vi "GetBlock.vi"(0 "error in":errorcluster, 2 "handle in":i16, 3 "Acquisition Settings":T3={"preTriggerSamples"=0, "postTriggerSamples"=1000, "timebase"=2, "Down-Sample Mode"=0, "Down Sample Ratio"=1} {"Down Sample Ratio" min=1 step=1; "Down-Sample Mode" items=["None"=0, "Aggregate"=1, "Decimate"=2, "Average"=4]}, 5 "enabled array":i16[](array[numeric])) -> (4 "overflow":i16, 6 "error IO":errorcluster, 7 "handle out":i16, 8 "noOfSamples":u32, 9 "Buffers (Max or non-aggregated)":T1, 10 "Min Buffers":T2)   [LabVIEW 2017]
doc: "This VI collects a block of data from the oscilloscope. This can be called in a loop in order to continually collect blocks of data. The oscilloscope should first be set up by using PicoScope3000aSettings.vi. The VI outputs data arrays in two clusters (max and min). If not using aggregation, 'Min Buffers' is not used."
uses:
  ps5000a.dll
panel:
  out "32bit integer":i32
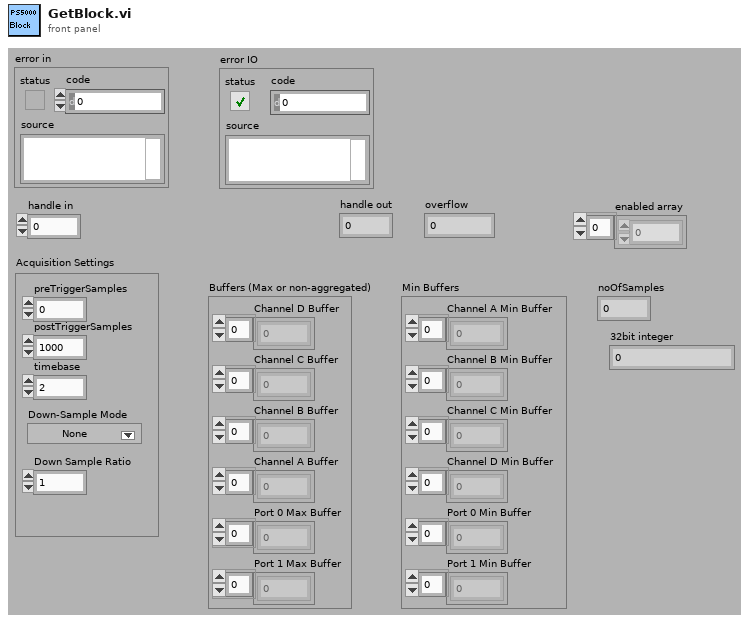
[diagram p1: front panel]
types:
  T1 = cluster{"Channel D Buffer":i16[], "Channel C Buffer":i16[], "Channel B Buffer":i16[], "Channel A Buffer":i16[], "Port 0 Max Buffer":i32[], "Port 1 Max Buffer":i32[]}
  T2 = cluster{"Channel A Min Buffer":i16[], "Channel B Min Buffer":i16[], "Channel C Min Buffer":i16[], "Channel D Min Buffer":i16[], "Port 0 Min Buffer":i32[], "Port 1 Min Buffer":i32[]}
  T3 = cluster{"preTriggerSamples":i32, "postTriggerSamples":i32, "timebase":u32, "Down-Sample Mode":u32, "Down Sample Ratio":u32}
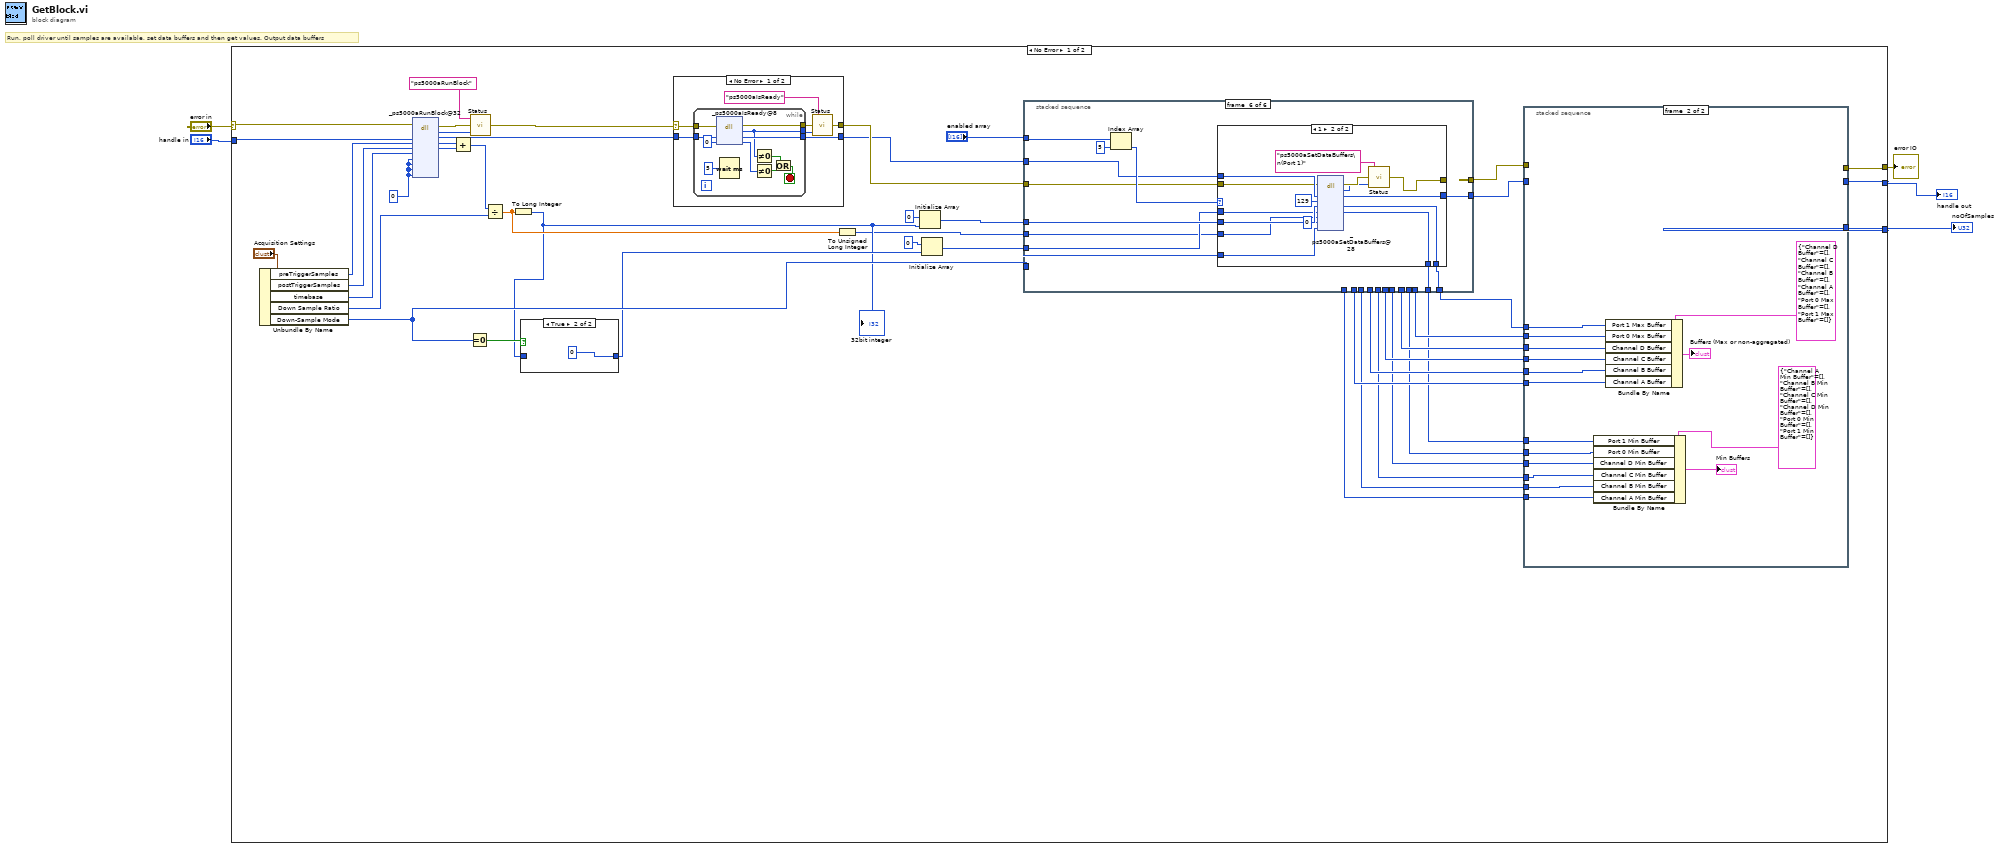
[diagram p0: block diagram]
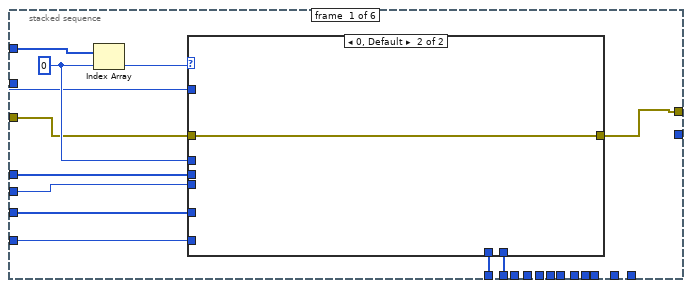
[diagram p3: hidden frame]
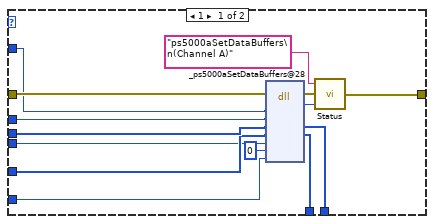
[diagram p4: hidden frame]
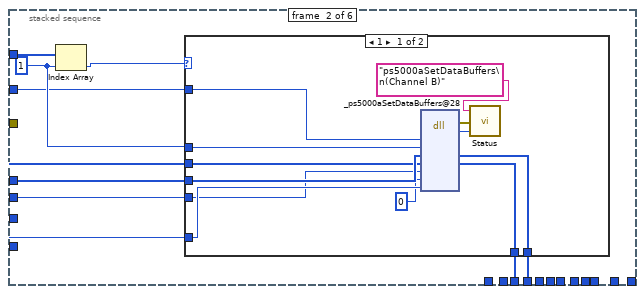
[diagram p5: hidden frame]
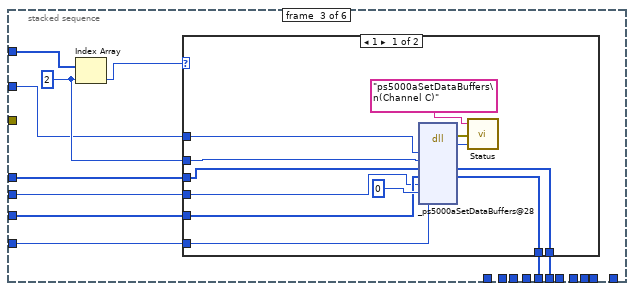
[diagram p7: hidden frame]
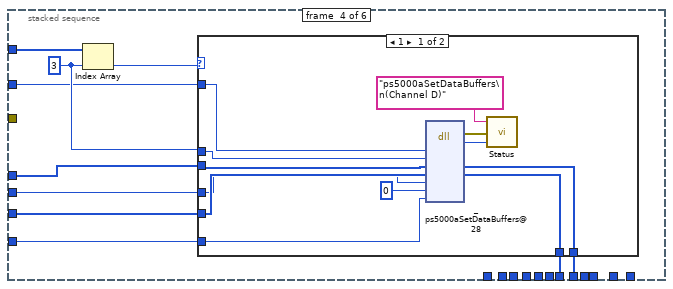
[diagram p9: hidden frame]
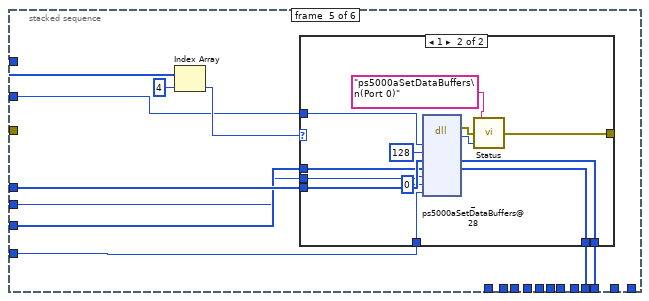
[diagram p11: hidden frame]
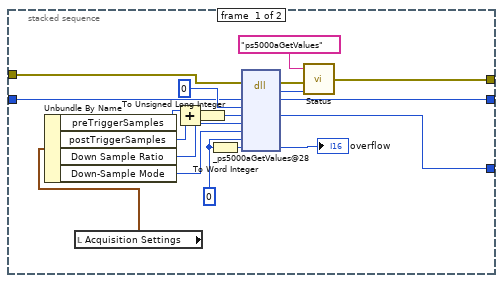
[diagram p14: hidden frame]
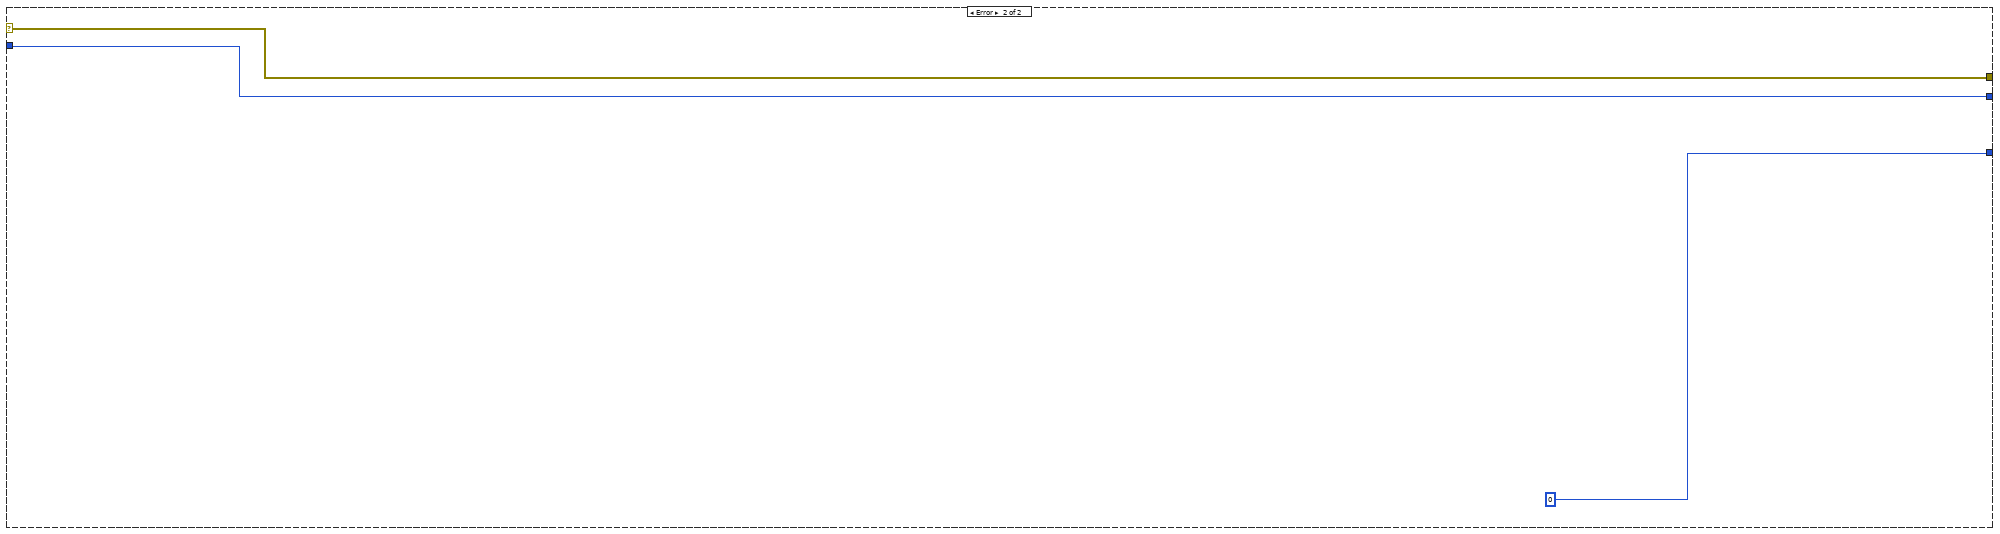
[diagram p16: hidden frame]
diagram:
  # "Run, poll driver until samples are available, set data buffers and then get values. Output data buffers"
  n1 = case shown="No Error" "error in" {
    selector: "error in" -> [w45 w255]
    tunnel: [w6 w255] -> w1
    tunnel: "handle in" -> [w44 w254]
    tunnel: [w43 w254] -> w5
    tunnel: [w36 u32 0 ("noOfSamples")] -> w2
    frame No Error {
      w40 = u32 0 ("pParameter")
      n2 = Unbundle By Name("Acquisition Settings") -> ("preTriggerSamples"=w39:i32, "postTriggerSamples"=w38:i32, "timebase"=w37:u32, "Down Sample Ratio"=w41:u32, "Down-Sample Mode"=w26:u32)
      n3 = dll-call lib="ps5000a.dll" fn="_ps5000aRunBlock@32" ("ps3000.dll:_ps3000_open_unit@0")(error in=w45, "handle"=w44, "preTriggerSamples"=w39, "postTriggerSamples"=w38, "timebase"=w37, "timeindisposed"=w40, "segmentIndex"=w40, "lpReady"=w40, "pParameter"=w40) -> (error out=w47:errorcluster, "PICO_STATUS"=w48:u32, "handle"=w35:i16, "preTriggerSamples"=w51:i32, "postTriggerSamples"=w50:i32)  [unwired: 7 in, 1 out]
      n4 = Add(x=w51, y=w50) -> (x+y=w42:i32)
      n5 = Equal To 0?(x=w26) -> (x = 0?=w24:bool)
      n6 = call "Status.vi"("PICO STATUS"=w48, "error in"=w47, "source"="ps5000aRunBlock") -> ("error out"=w7:errorcluster)
      n7 = Divide(x=w42, y=w41) -> (x/y=w27:dbl)
      n8 = To Long Integer(number=w27) -> (32bit integer=w23:i32)
      "32bit integer" <- w23
      n9 = case shown="True" w24 {
        tunnel: [w52 0] -> w25
        tunnel: w23 -> [w52 _]
        frame False {
        }
        frame True {
        }
      }
      n10 = case shown="No Error" w7 {
        selector: w7 -> [w237 w251]
        tunnel: w35 -> [w239 w252]
        tunnel: [w238 w252] -> w30
        tunnel: [w236 w251] -> w31
        frame No Error {
          n11 = while {
            tunnel: [w250] -> w238
            tunnel: w239 -> [w249]
            tunnel: [w244] -> w234
            tunnel: w237 -> [w243]
            tunnel: [w242] -> w235
            stop <- w248 stop-if-true
            n12 = dll-call lib="ps5000a.dll" fn="_ps5000aIsReady@8" ("ps3000.dll:_ps3000_open_unit@0")(error in=w243, "handle"=w249, "ready"=i16 0) -> (error out=w242:errorcluster, "PICO_STATUS"=w244:u32, "handle"=w250:i16, "ready"=w245:i16)  [unwired: 2 in, 1 out]
            n13 = Wait (ms)(milliseconds to wait=5) -> ()  [unwired: 1 out]
            n14 = Not Equal To 0?(x=w244) -> (x != 0?=w246:bool)
            n15 = Not Equal To 0?(x=w245) -> (x != 0?=w247:bool)
            n16 = Or(x=w246, y=w247) -> (x .or. y?=w248:bool)
          }
          n17 = call "Status.vi"("PICO STATUS"=w234, "error in"=w235, "source"="ps5000aIsReady") -> ("error out"=w236:errorcluster)
        }
        frame Error {
        }
      }
      n18 = To Unsigned Long Integer(number=w27) -> (unsigned 32bit integer=w9:u32)
      n19 = Initialize Array(i16 0 ("element"), w23) -> (w29:i16[])
      n20 = Initialize Array(i16 0 ("element"), w25) -> (w28:i16[])
      n21 = stacked-sequence {
        tunnel: "enabled array" -> [w64 w88 w111 w132 w156 w181]
        tunnel: w31 -> [w62 _ _ _ _ w170]
        tunnel: w30 -> [w61 w87 w109 w131 w153 w178]
        tunnel: w29 -> [w60 w86 w108 w130 w152 w177]
        tunnel: w28 -> [w59 w85 w107 w129 w151 w176]
        tunnel: w9 -> [w58 w83 w106 w128 w150 w175]
        tunnel: w26 -> [w57 w84 w105 w127 w149 w174]
        tunnel: [w56 _ _ _ _ _] -> w22
        tunnel: [w55 _ _ _ _ _] -> w21
        tunnel: [_ w82 _ _ _ _] -> w20
        tunnel: [_ w81 _ _ _ _] -> w19
        tunnel: [_ _ w104 _ _ _] -> w18
        tunnel: [_ _ w103 _ _ _] -> w17
        tunnel: [_ _ _ w126 _ _] -> w16
        tunnel: [_ _ _ w125 _ _] -> w15
        tunnel: [_ _ _ _ w148 _] -> w14
        tunnel: [_ _ _ _ w147 _] -> w13
        tunnel: [_ _ _ _ _ w173] -> w12
        tunnel: [_ _ _ _ _ w172] -> w11
        tunnel: [w54 _ _ _ _ _] -> w10
        tunnel: [_ _ _ _ _ w171] -> w8
        frame #0 {
          w65 = 0 ("dimension size")
          n22 = Index Array(array=w64, index=w65) -> (element=w63:i16)
          n23 = case shown="0, Default" w63 {
            tunnel: w65 -> [w74 _]
            tunnel: w62 -> [w79 w80]
            tunnel: w61 -> [w76 _]
            tunnel: w60 -> [w73 _]
            tunnel: w59 -> [w72 _]
            tunnel: w58 -> [w71 _]
            tunnel: w57 -> [w70 _]
            tunnel: [w68 _] -> w56
            tunnel: [w67 _] -> w55
            tunnel: [w66 w80] -> w54
            frame 1 {
              n24 = dll-call lib="ps5000a.dll" fn="_ps5000aSetDataBuffers@28" ("ps3000.dll:_ps3000_open_unit@0")(error in=w79, "handle"=w76, "channel"=w74, "bufferMax"=w73, "bufferMin"=w72, "bufferLth"=w71, "segmentIndex"=u32 0, "mode"=w70) -> (error out=w78:errorcluster, "PICO_STATUS"=w77:u32, "bufferMax"=w67:i16[], "bufferMin"=w68:i16[])  [unwired: 7 in, 1 out]
              n25 = call "Status.vi"("PICO STATUS"=w77, "error in"=w78, "source"="ps5000aSetDataBuffers\n(Channel A)") -> ("error out"=w66:errorcluster)
            }
            frame 0, Default {
            }
          }
        }
        frame #1 {
          w90 = 1 ("dimension size")
          n26 = Index Array(array=w88, index=w90) -> (element=w89:i16)
          n27 = case shown="1" w89 {
            tunnel: w90 -> [w99 _]
            tunnel: w87 -> [w98 _]
            tunnel: w86 -> [w97 _]
            tunnel: w85 -> [w96 _]
            tunnel: w84 -> [w95 _]
            tunnel: w83 -> [w93 _]
            tunnel: [w92 _] -> w82
            tunnel: [w91 _] -> w81
            frame 1 {
              n28 = dll-call lib="ps5000a.dll" fn="_ps5000aSetDataBuffers@28" ("ps3000.dll:_ps3000_open_unit@0")("handle"=w98, "channel"=w99, "bufferMax"=w97, "bufferMin"=w96, "bufferLth"=w93, "segmentIndex"=u32 0, "mode"=w95) -> (error out=w101:errorcluster, "PICO_STATUS"=w102:u32, "bufferMax"=w91:i16[], "bufferMin"=w92:i16[])  [unwired: 8 in, 1 out]
              n29 = call "Status.vi"("PICO STATUS"=w102, "error in"=w101, "source"="ps5000aSetDataBuffers\n(Channel B)") -> ()  [unwired: 1 out]
            }
            frame 0, Default {
            }
          }
        }
        frame #2 {
          w112 = 2 ("dimension size")
          n30 = Index Array(array=w111, index=w112) -> (element=w110:i16)
          n31 = case shown="1" w110 {
            tunnel: w112 -> [w120 _]
            tunnel: w109 -> [w119 _]
            tunnel: w108 -> [w118 _]
            tunnel: w107 -> [w117 _]
            tunnel: w106 -> [w116 _]
            tunnel: w105 -> [w115 _]
            tunnel: [w114 _] -> w104
            tunnel: [w113 _] -> w103
            frame 1 {
              n32 = dll-call lib="ps5000a.dll" fn="_ps5000aSetDataBuffers@28" ("ps3000.dll:_ps3000_open_unit@0")("handle"=w119, "channel"=w120, "bufferMax"=w118, "bufferMin"=w117, "bufferLth"=w116, "segmentIndex"=u32 0, "mode"=w115) -> (error out=w123:errorcluster, "PICO_STATUS"=w124:u32, "bufferMax"=w113:i16[], "bufferMin"=w114:i16[])  [unwired: 8 in, 1 out]
              n33 = call "Status.vi"("PICO STATUS"=w124, "error in"=w123, "source"="ps5000aSetDataBuffers\n(Channel C)") -> ()  [unwired: 1 out]
            }
            frame 0, Default {
            }
          }
        }
        frame #3 {
          w134 = 3 ("dimension size")
          n34 = Index Array(array=w132, index=w134) -> (element=w133:i16)
          n35 = case shown="1" w133 {
            tunnel: w134 -> [w142 _]
            tunnel: w131 -> [w141 _]
            tunnel: w130 -> [w140 _]
            tunnel: w129 -> [w139 _]
            tunnel: w128 -> [w138 _]
            tunnel: w127 -> [w137 _]
            tunnel: [w136 _] -> w126
            tunnel: [w135 _] -> w125
            frame 1 {
              n36 = dll-call lib="ps5000a.dll" fn="_ps5000aSetDataBuffers@28" ("ps3000.dll:_ps3000_open_unit@0")("handle"=w141, "channel"=w142, "bufferMax"=w140, "bufferMin"=w139, "bufferLth"=w138, "segmentIndex"=u32 0, "mode"=w137) -> (error out=w145:errorcluster, "PICO_STATUS"=w146:u32, "bufferMax"=w135:i16[], "bufferMin"=w136:i16[])  [unwired: 8 in, 1 out]
              n37 = call "Status.vi"("PICO STATUS"=w146, "error in"=w145, "source"="ps5000aSetDataBuffers\n(Channel D)") -> ()  [unwired: 1 out]
            }
            frame 0, Default {
            }
          }
        }
        frame #4 {
          n38 = Index Array(array=w156, index=4) -> (element=w154:i16)
          n39 = case shown="1" w154 {
            tunnel: w153 -> [_ w165]
            tunnel: w152 -> [_ w164]
            tunnel: w151 -> [_ w163]
            tunnel: w150 -> [_ w162]
            tunnel: w149 -> [_ w160]
            tunnel: [_ w159] -> w148
            tunnel: [_ w158] -> w147
            tunnel: [_ w157] -> _
            frame 0, Default {
            }
            frame 1 {
              n40 = dll-call lib="ps5000a.dll" fn="_ps5000aSetDataBuffers@28"("handle"=w165, "channel"=128, "bufferMax"=w164, "bufferMin"=w163, "bufferLth"=w162, "segmentIndex"=u32 0, "mode"=w160) -> (error out=w168:errorcluster, "PICO_STATUS"=w169:u32, "bufferMax"=w158:i16[], "bufferMin"=w159:i16[])  [unwired: 8 in, 1 out]
              n41 = call "Status.vi"("PICO STATUS"=w169, "error in"=w168, "source"="ps5000aSetDataBuffers\n(Port 0)") -> ("error out"=w157:errorcluster)
            }
          }
        }
        frame #5 {
          n42 = Index Array(array=w181, index=5) -> (element=w180:i16)
          n43 = case shown="1" w180 {
            tunnel: w178 -> [w182 w194]
            tunnel: w177 -> [_ w193]
            tunnel: w176 -> [_ w192]
            tunnel: w175 -> [_ w191]
            tunnel: w174 -> [_ w189]
            tunnel: [_ w188] -> w173
            tunnel: [_ w187] -> w172
            tunnel: [_ w184] -> _
            tunnel: [w182 w185] -> w171
            tunnel: w170 -> [_ w183]
            frame 0, Default {
            }
            frame 1 {
              n44 = dll-call lib="ps5000a.dll" fn="_ps5000aSetDataBuffers@28" ("ps3000.dll:_ps3000_open_unit@0")(error in=w183, "handle"=w194, "channel"=129, "bufferMax"=w193, "bufferMin"=w192, "bufferLth"=w191, "segmentIndex"=u32 0, "mode"=w189) -> (error out=w197:errorcluster, "PICO_STATUS"=w186:u32, "handle"=w185:i16, "bufferMax"=w187:i16[], "bufferMin"=w188:i16[])  [unwired: 6 in, 1 out]
              n45 = call "Status.vi"("PICO STATUS"=w186, "error in"=w197, "source"="ps5000aSetDataBuffers\n(Port 1)") -> ("error out"=w184:errorcluster)
            }
          }
        }
      }
      n46 = stacked-sequence {
        tunnel: [w211 _] -> w43
        tunnel: [w201 _] -> w36
        tunnel: w22 -> [_ w228]
        tunnel: w21 -> [_ w227]
        tunnel: w20 -> [_ w226]
        tunnel: w19 -> [_ w225]
        tunnel: w18 -> [_ w223]
        tunnel: w17 -> [_ w224]
        tunnel: w16 -> [_ w222]
        tunnel: w15 -> [_ w221]
        tunnel: w14 -> [_ w220]
        tunnel: w13 -> [_ w219]
        tunnel: w12 -> [_ w218]
        tunnel: w11 -> [_ w217]
        tunnel: w10 -> [w200 _]
        tunnel: w8 -> [w199 _]
        tunnel: [w198 _] -> w6
        frame #0 {
          w215 = u32 0 ("overflow")
          n47 = local read "Acquisition Settings"() -> (w209:T3)
          n48 = Unbundle By Name(w209) -> ("preTriggerSamples"=w206:i32, "postTriggerSamples"=w207:i32, "Down Sample Ratio"=w208:u32, "Down-Sample Mode"=w204:u32)
          n49 = Add(x=w206, y=w207) -> (x+y=w205:i32)
          n50 = To Unsigned Long Integer(number=w205) -> (unsigned 32bit integer=w203:u32)
          n51 = To Word Integer(number=w215) -> (16bit integer=w202:i16)
          n52 = dll-call lib="ps5000a.dll" fn="_ps5000aGetValues@28" ("ps3000.dll:_ps3000_open_unit@0")(error in=w200, "handle"=w199, "startIndex"=u32 0, "noOfSamples"=w203, "downSampleRatio"=w208, "downSampleRatioMode"=w204, "segmentIndex"=w215, "overflow"=w202) -> (error out=w213:errorcluster, "PICO_STATUS"=w214:u32, "handle"=w211:i16, "noOfSamples"=w201:u32, "overflow"=→"overflow":i16)  [unwired: 6 in, 1 out]
          n53 = call "Status.vi"("PICO STATUS"=w214, "error in"=w213, "source"="ps5000aGetValues") -> ("error out"=w198:errorcluster)
        }
        frame #1 {
          n54 = Bundle By Name(cluster=T2 {"Channel A Min Buffer"=[], "Channel B Min Buffer"=[], "Channel C Min Buffer"=[], "Channel D Min Buffer"=[], "Port 0 Min Buffer"=[], "Port 1 Min Buffer"=[]} ("Min Buffers"), "Port 1 Min Buffer"=w218, "Port 0 Min Buffer"=w220, "Channel D Min Buffer"=w222, "Channel C Min Buffer"=w223, "Channel B Min Buffer"=w226, "Channel A Min Buffer"=w228) -> (→"Min Buffers":T2)
          n55 = Bundle By Name(cluster=T1 {"Channel D Buffer"=[], "Channel C Buffer"=[], "Channel B Buffer"=[], "Channel A Buffer"=[], "Port 0 Max Buffer"=[], "Port 1 Max Buffer"=[]} ("Buffers (Max or non-aggregated)"), "Port 1 Max Buffer"=w217, "Port 0 Max Buffer"=w219, "Channel D Buffer"=w221, "Channel C Buffer"=w224, "Channel B Buffer"=w225, "Channel A Buffer"=w227) -> (→"Buffers (Max or non-aggregated)":T1)
        }
      }
    }
    frame Error {
    }
  }
  "handle out" <- w5
  "noOfSamples" <- w2
  "error IO" <- w1
